vi "Property Tree Set Value_Remove Items_old.vi"(8 "Error In":errorcluster, 9 "Tag Selected":string[](array[string]), 10 "Active Tree":refnum<vi>, 11 "All Tree Refs":refnum<vi>[](array[refnum])) -> (0 "Error Out":errorcluster)   [LabVIEW 2023]
doc: "Toggle has already happened, so here we determine if row is selecgted and deal with updating the tree value"
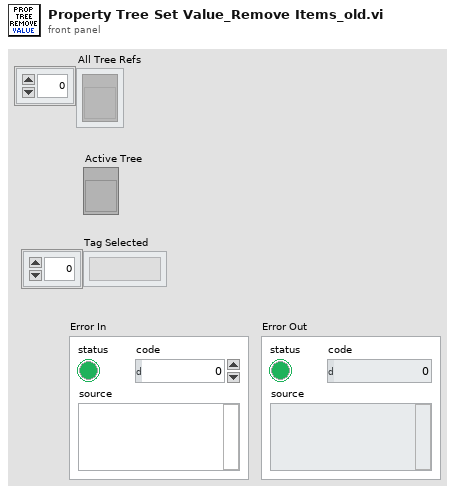
[diagram p1: front panel]
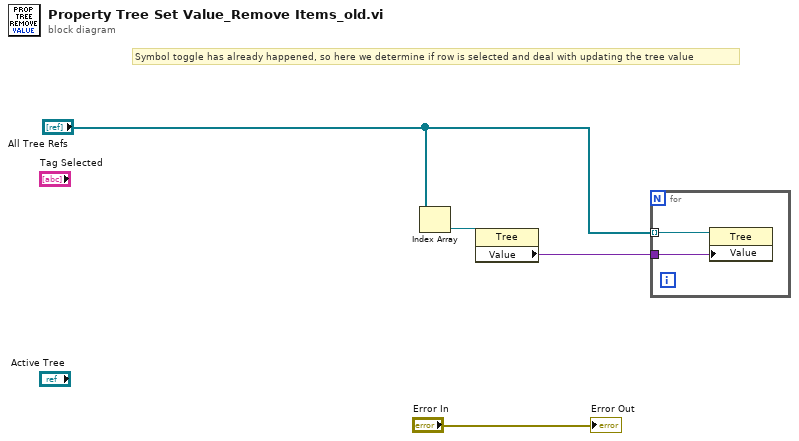
[diagram p0: block diagram]
diagram:
  # "Symbol toggle has already happened, so here we determine if row is selected and deal with updating the tree value"
  n1 = Index Array(array="All Tree Refs") -> (element=w2:refnum<vi>)  [unwired: 1 in]
  n2 = property class="Tree"(reference=w2) -> ("Value"=w1:variant)  [unwired: 1 in, 2 out]
  n3 = for {
    tunnel: w1 -> [w5]
    tunnel: "All Tree Refs" -> [w6] mode=indexing
    n4 = property class="Tree"(reference=w6, "Value"=w5) -> ()  [unwired: 1 in, 2 out]
  }
  "Error Out" <- "Error In"
